vi "CREATE_INITIAL_STRING.vi"(9 "appended array":string[](array[string]), 11 "String in":string) -> (3 "String out":string)   [LabVIEW 2016]
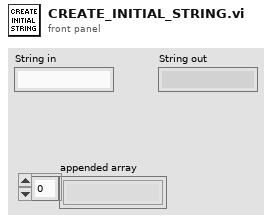
[diagram p1: front panel]
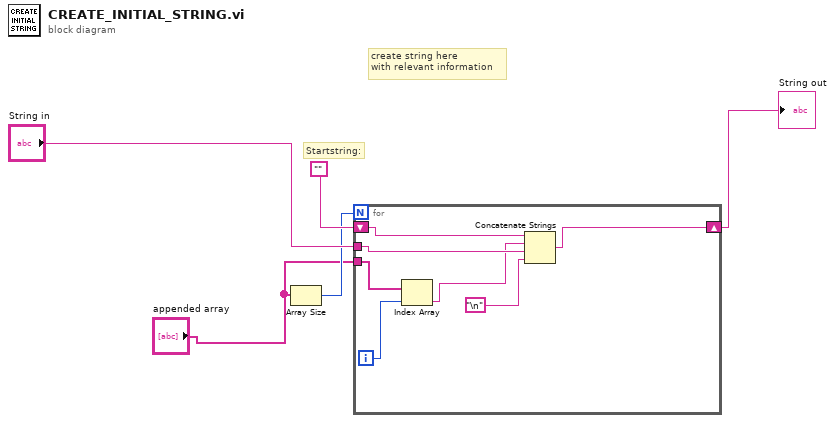
[diagram p0: block diagram]
diagram:
  # "Startstring:"
  # "create string here \nwith relevant information"
  n1 = Array Size(array="appended array") -> (size(s)=w2:i32)
  n2 = for {
    N: w2 -> [_]
    tunnel: "appended array" -> [w11]
    tunnel: "String in" -> [w10]
    shift-right: [w8] -> w5
    shift-left: "" -> [w9]
    i -> [w12]
    n3 = Index Array(array=w11, index=w12) -> (element=w7:string)
    n4 = Concatenate Strings(w9, w7, w10, "\n" ("End of Line Constant")) -> (w8:string)
  }
  "String out" <- w5
